vi "10转16.vi"(2 "错误In":errorcluster, 3 "字符串":string) -> (0 "错误Out":errorcluster, 1 "字符串 2":string)   [LabVIEW 2015]
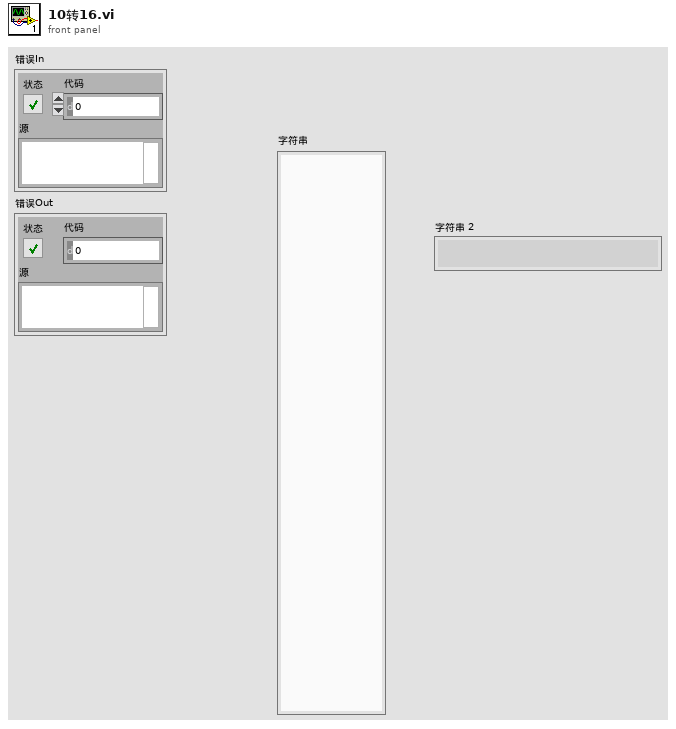
[diagram p1: front panel]
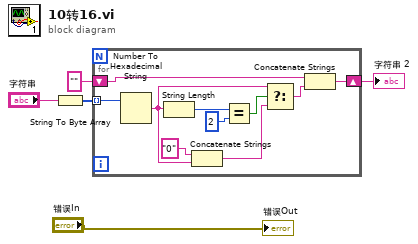
[diagram p0: block diagram]
diagram:
  n1 = String To Byte Array(string="字符串") -> (unsigned byte array=w4:u8[])
  n2 = for {
    tunnel: w4 -> [w13] mode=indexing
    shift-right: [w15] -> w2
    shift-left: "" ("字符串") -> [w14]
    n3 = Number To Hexadecimal String(2:w13) -> (0:w6:string)  [unwired: 1 in]
    n4 = String Length(string=w6) -> (length=w9:i32)
    n5 = Concatenate Strings("0" ("字符串"), w6) -> (w10:string)
    n6 = Equal?(x=w9, y=2) -> (x = y?=w8:bool)
    n7 = Select(t=w6, s=w8, f=w10) -> (s? t:f=w11:string)
    n8 = Concatenate Strings(w14, w11) -> (w15:string)
  }
  "字符串 2" <- w2
  "错误Out" <- "错误In"
